vi "Current Lamps.vi"(8 "Dome Percent":i8=70 caption="%" min=0 max=100 step=1, 9 "Quartz Intensity":i8=70 caption="%" min=0 max=100 step=1, 10 "Dome":bool, 11 "Lamp Cluster":T1) -> (3 "Current Lamps":string)   [LabVIEW 2015]
panel:
  out "Quartz Actual":i8 caption="%"
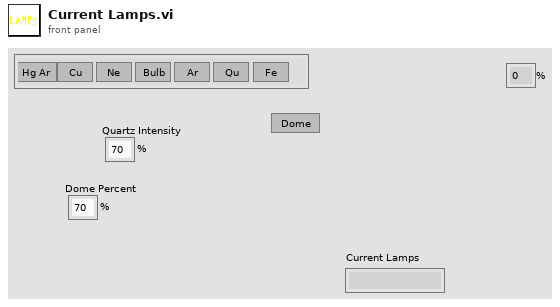
[diagram p1: front panel]
types:
  T1 = cluster{"Hg(Ar)":bool, "Cu":bool, "Ne":bool, "Ar":bool, "Quartz":bool, "Fe":bool, "Bulb":bool}
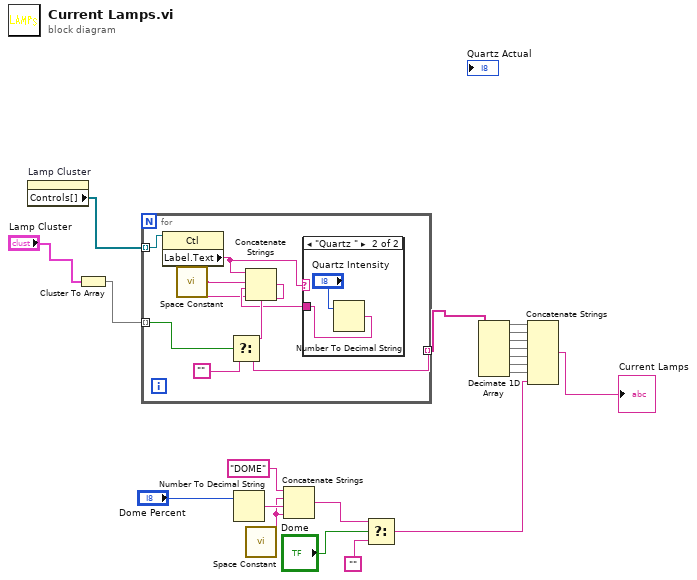
[diagram p0: block diagram]
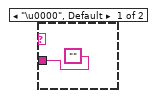
[diagram p2: hidden frame]
diagram:
  n1 = property on="Lamp Cluster" class="Clust (strict)"() -> ("Controls[]"=w19:refnum<vi>[])  [unwired: 2 in, 2 out]
  n2 = Cluster To Array(cluster="Lamp Cluster") -> (array=w18:bool[])
  n3 = for {
    tunnel: w19 -> [w27] mode=indexing
    tunnel: w18 -> [w26] mode=indexing
    tunnel: [w24] -> w17 mode=indexing
    n4 = property on="Property Node" class="Ctl"(reference=w27) -> ("Label.Text"=w23:string)  [unwired: 1 in, 2 out]
    n5 = call <vilib>:"Space Constant.vi"() -> ("String"=w21:string)
    n6 = case shown="\"Quartz \"" w23 {
      tunnel: ["" w30] -> w22
      frame "\u0000", Default {
      }
      frame "Quartz " {
        n7 = Number To Decimal String(number="Quartz Intensity") -> (decimal integer string=w30:string)  [unwired: 1 in]
      }
    }
    n8 = Concatenate Strings(w23, w21, w22, w21) -> (w25:string)
    n9 = Select(t=w25, s=w26, f="") -> (s? t:f=w24:string)
  }
  n10 = Number To Decimal String(number="Dome Percent") -> (decimal integer string=w4:string)  [unwired: 1 in]
  n11 = call <vilib>:"Space Constant.vi"() -> ("String"=w3:string)
  n12 = Concatenate Strings("DOME", w3, w4, w3) -> (w2:string)
  n13 = Select(t=w2, s="Dome", f="") -> (s? t:f=w1:string)
  n14 = Decimate 1D Array(w17) -> (w16:string[], w15:string[], w14:string[], w13:string[], w12:string[], w11:string[], w10:string[])
  n15 = Concatenate Strings(w16, w15, w14, w13, w12, w11, w10, w1) -> (→"Current Lamps":string)
